vi "RotateVector.vi"(10 "Angle (Degrees)":dbl, 11 "Vector":cluster{dbl, dbl}) -> (3 "Rotated Vector":cluster{dbl, dbl})   [LabVIEW 2020]
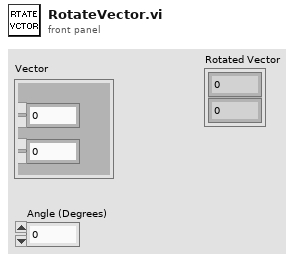
[diagram p1: front panel]
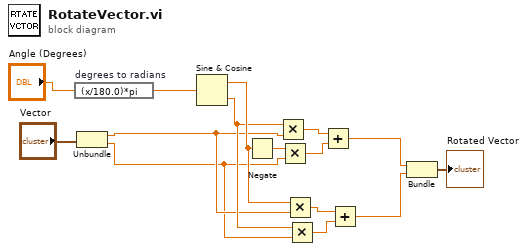
[diagram p0: block diagram]
diagram:
  n1 = expression code="(x/180.0)*pi" "degrees to radians"("Angle (Degrees)") -> (w11:dbl)
  n2 = Unbundle("Vector") -> (w5:dbl, w4:dbl)
  n3 = Sine & Cosine(0:w11) -> (1:w9:dbl, 2:w8:dbl)
  n4 = Negate(x=w9) -> (-x=w10:dbl)
  n5 = Multiply(x=w8, y=w5) -> (x*y=w15:dbl)
  n6 = Multiply(x=w10, y=w4) -> (x*y=w14:dbl)
  n7 = Multiply(x=w9, y=w5) -> (x*y=w13:dbl)
  n8 = Multiply(x=w8, y=w4) -> (x*y=w12:dbl)
  n9 = Add(x=w15, y=w14) -> (x+y=w3:dbl)
  n10 = Add(x=w13, y=w12) -> (x+y=w2:dbl)
  n11 = Bundle(w3, w2) -> (→"Rotated Vector":cluster{dbl, dbl})  [unwired: 1 in]
